vi "CREATE RENTED ITEM SQL QUERY.vi"(0 "What to Search":string, 5 "Search Column Name":string, 7 "Sorting Column Name":string, 9 "Column to Search In":u16, 12 "Date Range":u16(ring) items=["Greater Than", "Less Than", "Between"], 13 "Dates Less Than":string="8/1/2023", 14 "Dates Greater Than":string="8/1/2023") -> (4 "SQL QUERY":string)   [LabVIEW 2019]
panel:
  in  "Column to Sort By":u16
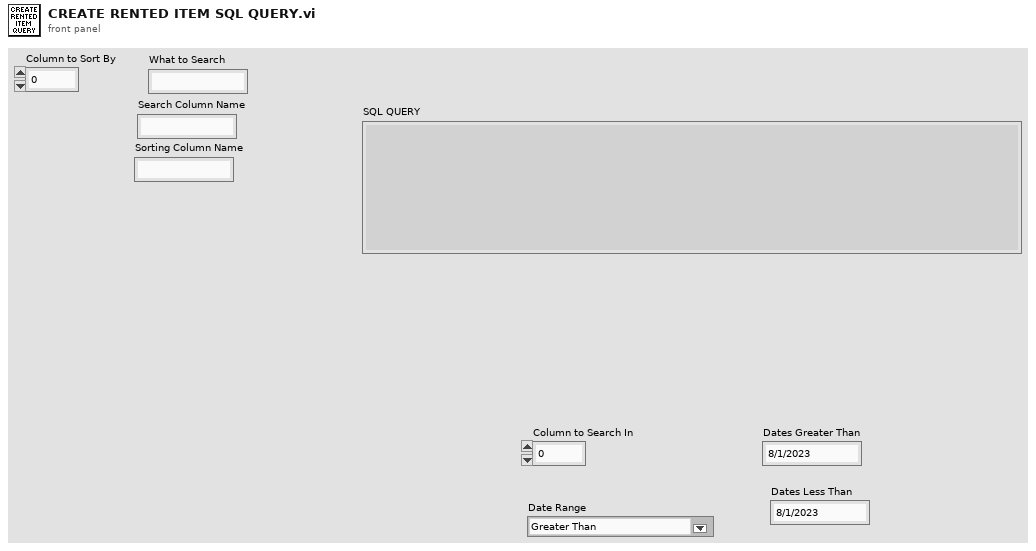
[diagram p1: front panel]
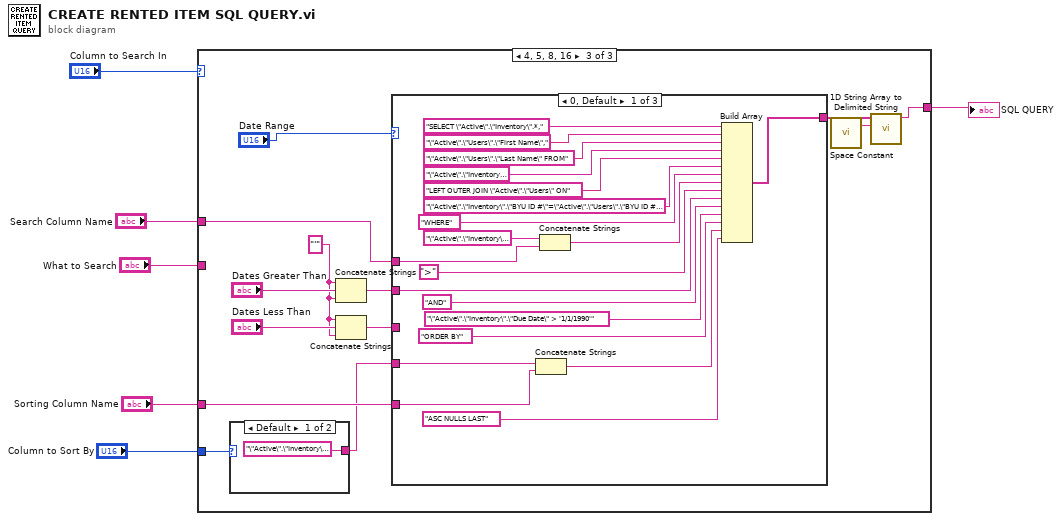
[diagram p0: block diagram]
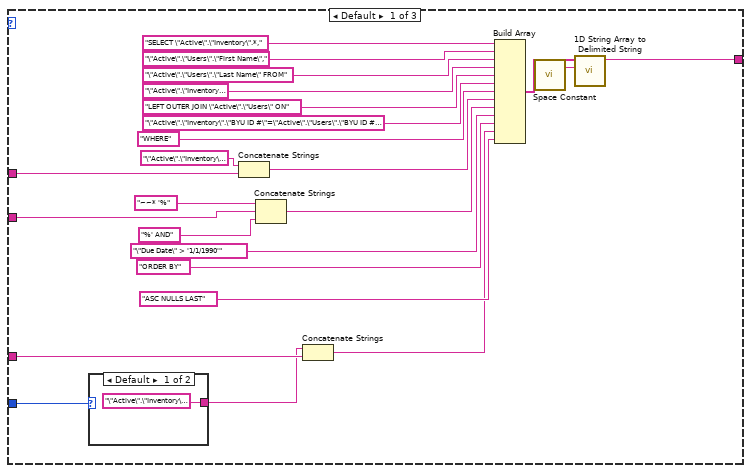
[diagram p2: hidden frame]
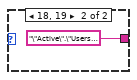
[diagram p3: hidden frame]
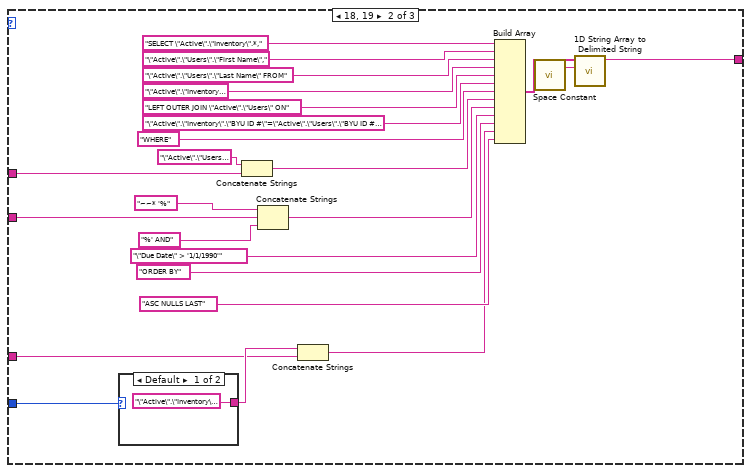
[diagram p4: hidden frame]
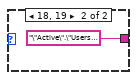
[diagram p5: hidden frame]
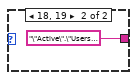
[diagram p6: hidden frame]
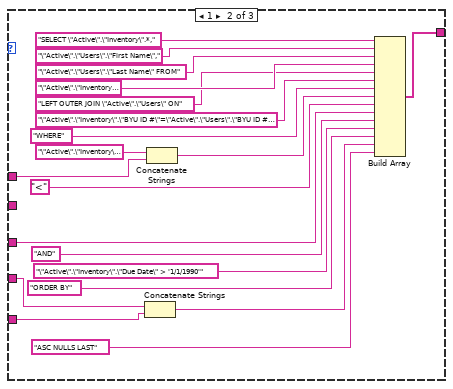
[diagram p7: hidden frame]
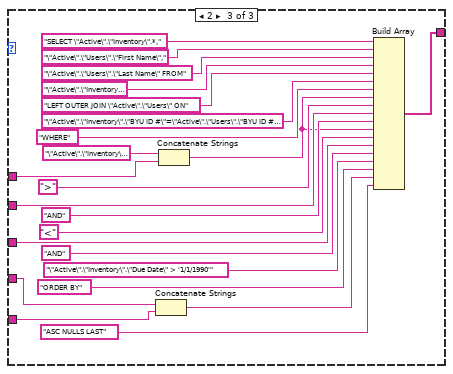
[diagram p8: hidden frame]
diagram:
  n1 = case shown="4, 5, 8, 16" "Column to Search In" {
    tunnel: "Sorting Column Name" -> [w9 w34 w69]
    tunnel: "Search Column Name" -> [w13 w37 w70]
    tunnel: [w15 w41 w66] -> w3
    tunnel: "What to Search" -> [w14 w40 _]
    tunnel: "Column to Sort By" -> [w10 w39 w60]
    frame Default {
      n2 = case shown="Default" w10 {
        tunnel: ["\"Active\".\"Inventory\"." ("string") "\"Active\".\"Users\"." ("string")] -> w8
        frame Default {
        }
        frame 18, 19 {
        }
      }
      n3 = Concatenate Strings("\"Active\".\"Inventory\"." ("string"), w13) -> (w11:string)
      n4 = Concatenate Strings("~~* '%" ("string"), w14, "%' AND" ("string")) -> (w26:string)
      n5 = Concatenate Strings(w8, w9) -> (w7:string)
      n6 = Build Array("SELECT \"Active\".\"Inventory\".*," ("string"), "\"Active\".\"Users\".\"First Name\"," ("string"), "\"Active\".\"Users\".\"Last Name\" FROM" ("string"), "\"Active\".\"Inventory\"" ("string"), "LEFT OUTER JOIN \"Active\".\"Users\" ON" ("string"), "\"Active\".\"Inventory\".\"BYU ID #\"=\"Active\".\"Users\".\"BYU ID #\"" ("string"), "WHERE" ("string"), w11, w26, "\"Due Date\" > '1/1/1990'" ("string"), "ORDER BY" ("string"), w7, "ASC NULLS LAST" ("string")) -> (w29:string[])
      n7 = call <vilib>:"Space Constant.vi"() -> ("String"=w30:string)
      n8 = call <vilib>:"1D String Array to Delimited String.vi"("delimiter"=w30, "string array"=w29) -> ("delimited string"=w15:string)  [unwired: 9 in]
    }
    frame 18, 19 {
      n9 = case shown="Default" w39 {
        tunnel: ["\"Active\".\"Inventory\"." ("string") "\"Active\".\"Users\"." ("string")] -> w35
        frame Default {
        }
        frame 18, 19 {
        }
      }
      n10 = Concatenate Strings("\"Active\".\"Users\"." ("string"), w37) -> (w36:string)
      n11 = Concatenate Strings("~~* '%" ("string"), w40, "%' AND" ("string")) -> (w52:string)
      n12 = Concatenate Strings(w35, w34) -> (w33:string)
      n13 = Build Array("SELECT \"Active\".\"Inventory\".*," ("string"), "\"Active\".\"Users\".\"First Name\"," ("string"), "\"Active\".\"Users\".\"Last Name\" FROM" ("string"), "\"Active\".\"Inventory\"" ("string"), "LEFT OUTER JOIN \"Active\".\"Users\" ON" ("string"), "\"Active\".\"Inventory\".\"BYU ID #\"=\"Active\".\"Users\".\"BYU ID #\"" ("string"), "WHERE" ("string"), w36, w52, "\"Due Date\" > '1/1/1990'" ("string"), "ORDER BY" ("string"), w33, "ASC NULLS LAST" ("string")) -> (w55:string[])
      n14 = call <vilib>:"Space Constant.vi"() -> ("String"=w56:string)
      n15 = call <vilib>:"1D String Array to Delimited String.vi"("delimiter"=w56, "string array"=w55) -> ("delimited string"=w41:string)  [unwired: 9 in]
    }
    frame 4, 5, 8, 16 {
      w61 = "'"
      n16 = case shown="Default" w60 {
        tunnel: ["\"Active\".\"Inventory\"." ("string") "\"Active\".\"Users\"." ("string")] -> w59
        frame Default {
        }
        frame 18, 19 {
        }
      }
      n17 = Concatenate Strings(w61, "Dates Greater Than", w61) -> (w64:string)
      n18 = Concatenate Strings(w61, "Dates Less Than", w61) -> (w65:string)
      n19 = case shown="0, Default" "Date Range" {
        tunnel: w70 -> [w87 w105 w129]
        tunnel: w64 -> [w84 _ w126]
        tunnel: w69 -> [w78 w98 w118]
        tunnel: w65 -> [_ w102 w122]
        tunnel: [w75 w95 w115] -> w67
        tunnel: w59 -> [w74 w94 w114]
        frame 0, Default {
          n20 = Concatenate Strings(w74, w78) -> (w77:string)
          n21 = Concatenate Strings("\"Active\".\"Inventory\"." ("string"), w87) -> (w86:string)
          n22 = Build Array("SELECT \"Active\".\"Inventory\".*," ("string"), "\"Active\".\"Users\".\"First Name\"," ("string"), "\"Active\".\"Users\".\"Last Name\" FROM" ("string"), "\"Active\".\"Inventory\"" ("string"), "LEFT OUTER JOIN \"Active\".\"Users\" ON" ("string"), "\"Active\".\"Inventory\".\"BYU ID #\"=\"Active\".\"Users\".\"BYU ID #\"" ("string"), "WHERE" ("string"), w86, ">" ("string"), w84, "AND" ("string"), "\"Active\".\"Inventory\".\"Due Date\" > '1/1/1990'" ("string"), "ORDER BY" ("string"), w77, "ASC NULLS LAST" ("string")) -> (w75:string[])
        }
        frame 1 {
          n23 = Concatenate Strings(w94, w98) -> (w97:string)
          n24 = Concatenate Strings("\"Active\".\"Inventory\"." ("string"), w105) -> (w104:string)
          n25 = Build Array("SELECT \"Active\".\"Inventory\".*," ("string"), "\"Active\".\"Users\".\"First Name\"," ("string"), "\"Active\".\"Users\".\"Last Name\" FROM" ("string"), "\"Active\".\"Inventory\"" ("string"), "LEFT OUTER JOIN \"Active\".\"Users\" ON" ("string"), "\"Active\".\"Inventory\".\"BYU ID #\"=\"Active\".\"Users\".\"BYU ID #\"" ("string"), "WHERE" ("string"), w104, "<" ("string"), w102, "AND" ("string"), "\"Active\".\"Inventory\".\"Due Date\" > '1/1/1990'" ("string"), "ORDER BY" ("string"), w97, "ASC NULLS LAST" ("string")) -> (w95:string[])
        }
        frame 2 {
          n26 = Concatenate Strings(w114, w118) -> (w117:string)
          n27 = Concatenate Strings("\"Active\".\"Inventory\"." ("string"), w129) -> (w124:string)
          n28 = Build Array("SELECT \"Active\".\"Inventory\".*," ("string"), "\"Active\".\"Users\".\"First Name\"," ("string"), "\"Active\".\"Users\".\"Last Name\" FROM" ("string"), "\"Active\".\"Inventory\"" ("string"), "LEFT OUTER JOIN \"Active\".\"Users\" ON" ("string"), "\"Active\".\"Inventory\".\"BYU ID #\"=\"Active\".\"Users\".\"BYU ID #\"" ("string"), "WHERE" ("string"), w124, ">" ("string"), w126, "AND" ("string"), w124, "<" ("string"), w122, "AND" ("string"), "\"Active\".\"Inventory\".\"Due Date\" > '1/1/1990'" ("string"), "ORDER BY" ("string"), w117, "ASC NULLS LAST" ("string")) -> (w115:string[])
        }
      }
      n29 = call <vilib>:"Space Constant.vi"() -> ("String"=w68:string)
      n30 = call <vilib>:"1D String Array to Delimited String.vi"("delimiter"=w68, "string array"=w67) -> ("delimited string"=w66:string)  [unwired: 9 in]
    }
  }
  "SQL QUERY" <- w3
